vi "Test Temperature.vi"(8 "error in (no error)":errorcluster, 11 "Instrument.Cryostat in":refnum<class "Instrument.Cryostat.lvclass">) -> (0 "error out":errorcluster, 3 "Instrument.Cryostat out":refnum<class "Instrument.Cryostat.lvclass">)   [LabVIEW 2019]
uses:
  lvsrc/Instrument Types/Cryostat/Instrument.Cryostat.lvclass
  <vilib>/addons/_JKI Toolkits/Caraya/classes/Assert/Assert Error.vi
  <vilib>/addons/_JKI Toolkits/Caraya/classes/Assert/Assert Almost Equal_Float.vi
  <vilib>/addons/_JKI Toolkits/Caraya/classes/Test/Test.lvclass
  <vilib>/addons/_JKI Toolkits/Caraya/classes/Assert/Assert.lvclass
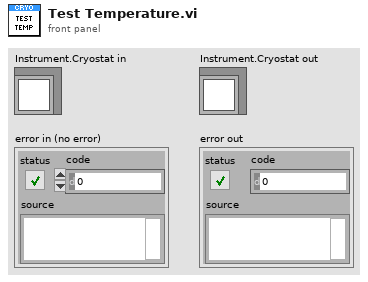
[diagram p1: front panel]
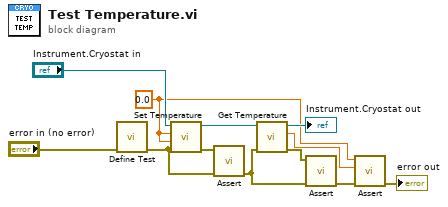
[diagram p0: block diagram]
diagram:
  w1 = 0.0 ("Angle (°)")
  n1 = call <vilib>:"Define Test.vi"("error in (no error)"="error in (no error)") -> ("error out"=w6:errorcluster)  [unwired: 10 in]
  n2 = call-dynamic "Set Temperature.vi"("error in (no error)"=w6, "Rate (K/min)"=w1, "Temperature (K)"=w1, "Instrument.Cryostat in"="Instrument.Cryostat in") -> ("error out"=w5:errorcluster, "Instrument.Cryostat out"=w9:refnum<class "Instrument.Cryostat.lvclass">)  [unwired: 6 in]
  n3 = call-poly <vilib>:"Assert.vi"("error in (no error)"=w6, "Error?"=w5) -> ("error out"=w4:errorcluster)  [unwired: 9 in]
  n4 = call-dynamic "Get Temperature.vi"("error in (no error)"=w4, "Instrument.Cryostat in"=w9) -> ("error out"=w3:errorcluster, "Temperature (K)"=w2:dbl, "Instrument.Cryostat out"=→"Instrument.Cryostat out":refnum<class "Instrument.Cryostat.lvclass">)  [unwired: 5 in, 2 out]
  n5 = call-poly <vilib>:"Assert.vi"("error in (no error)"=w4, "Error?"=w3) -> ("error out"=w11:errorcluster)  [unwired: 9 in]
  n6 = call-poly <vilib>:"Assert.vi"("error in (no error)"=w11, "Y"=w2, "X"=w1) -> ("error out"=→"error out":errorcluster)  [unwired: 8 in]
